vi "PH_USB600x_AnalogReader.evt call set timing mode.vi"(0 "i ref in":refnum<vi>, 2 "Instance":string, 3 "Timing":T1={"Samples per Channel"=1000, "Rate"=1000.0} {"Rate" format="%0.2f"; "Samples per Channel" min=1}, 5 "error in":errorcluster) -> (14 "i ref out":refnum<vi>, 19 "error out":errorcluster)   [LabVIEW 2014, in "PH_USB600x_AnalogReader.lvlib"]
doc: "This VI sends a simple event call."
uses:
  PH_USB600x_AnalogReader.lvlib
  PH_USB600x_AnalogReader.Timing.ctl
  CSCore/CSSystem/CoreLib/CoreLib.int 2 byte array.vi
  CSCore/CSSystem/CoreLib/CoreLib.double 2 byte array.vi
  CSCore/BaseProcess/BaseProcess.lvlib
  CSCore/CSSystem/CoreLib/CoreLib.lvlib
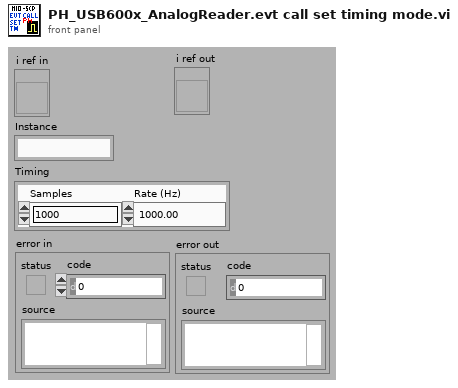
[diagram p1: front panel]
types:
  T1 = typedef "PH_USB600x_AnalogReader.lvlib/PH_USB600x_AnalogReader.Timing.ctl" = cluster{"Samples per Channel":i32, "Rate":dbl}
  T2 = typedef "CoreDefs.rawDataType.ctl" = i8[]
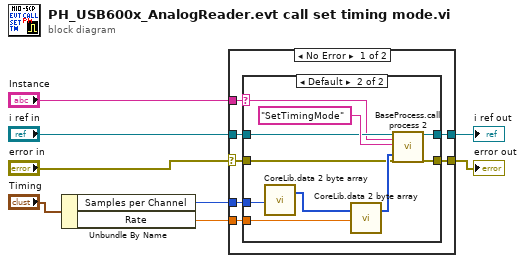
[diagram p0: block diagram]
diagram:
  n1 = Unbundle By Name("Timing") -> ("Samples per Channel"=w2:i32, "Rate"=w1:dbl)
  n2 = case shown="No Error" "error in" {
    selector: "error in" -> [w11 w28]
    tunnel: "Instance" -> [w10 _]
    tunnel: "i ref in" -> [w15 w29]
    tunnel: w1 -> [w14 _]
    tunnel: [w13 w29] -> w6
    tunnel: [w12 w28] -> w5
    tunnel: w2 -> [w9 _]
    frame No Error {
      n3 = case shown="Default" w10 {
        selector: w10 -> [_ w20]
        tunnel: w15 -> [w16 w26]
        tunnel: w14 -> [_ w24]
        tunnel: [w16 w23] -> w13
        tunnel: [w17 w22] -> w12
        tunnel: w11 -> [w17 w21]
        tunnel: w9 -> [_ w18]
        frame "", "N/A" {
        }
        frame Default {
          n4 = call-poly "CoreLib.data 2 byte array.vi"("i32"=w18) -> ("byteArray out"=w19:T2)  [unwired: 18 in]
          n5 = call-poly "CoreLib.data 2 byte array.vi"("byteArray"=w19, "f64"=w24) -> ("byteArray out"=w25:T2)  [unwired: 17 in]
          n6 = call "BaseProcess.call process 2.vi"("i ref in"=w26, "Object"=w20, "Selector"="SetTimingMode", "Data"=w25, "error in (no error)"=w21) -> ("i ref out"=w23:refnum<vi>, "error out"=w22:errorcluster)  [unwired: 13 in]
        }
      }
    }
    frame Error {
    }
  }
  "i ref out" <- w6
  "error out" <- w5
